vi "Pcre2MatchContextFree8.vi"(8 "error in":errorcluster, 11 "pMatchContext":u64 format="%.0x") -> (0 "error out":errorcluster)   [LabVIEW 2021, in "libpcre2-8.lvlib"]
uses:
  libpcre2-8.lvlib
  libpcre2-8-x32.dll
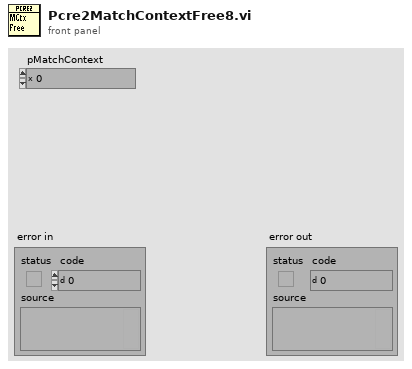
[diagram p1: front panel]
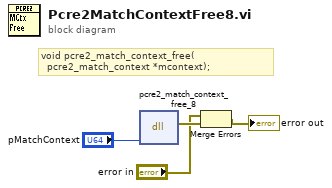
[diagram p0: block diagram]
diagram:
  # "void pcre2_match_context_free(\n  pcre2_match_context *mcontext);"
  n1 = dll-call lib="libpcre2-8-x*.dll" fn="pcre2_match_context_free_8"("mcontext"="pMatchContext") -> (error out=w3:errorcluster)  [unwired: 5 in, 1 out]
  n2 = Merge Errors("error in", w3) -> (→"error out":errorcluster)
